vi "Write frame.vi"(8 "error in (no error)":errorcluster, 10 "frame":T1, 11 "Ephemeris in":refnum<class "Ephemeris.lvclass">) -> (0 "error out":errorcluster, 3 "Ephemeris out":refnum<class "Ephemeris.lvclass">)   [LabVIEW 2022 SP3, in "TCSDataDefinitions.lvlib" / "TCSCommand.lvlib" / "TargetConfiguration.lvlib" / "Target.lvlib" / "Ephemeris.lvclass"]
uses:
  Ephemeris.lvclass
  FixedTarget/Enumerations/FrameValues.ctl
  Ephemeris.lvclass/Ephemeris.ctl
  FixedTarget/FixedTarget.lvlib
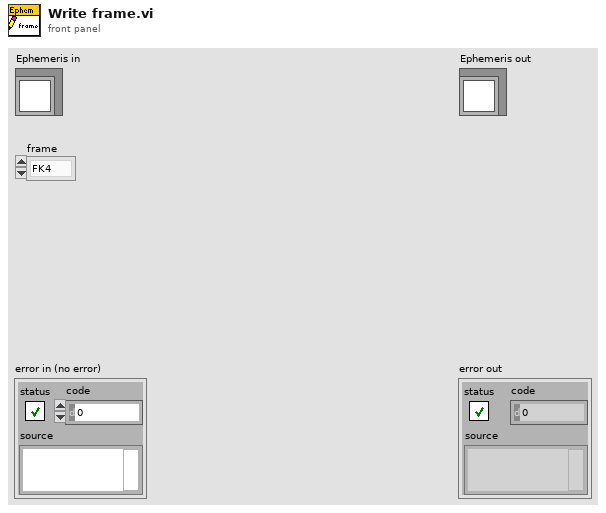
[diagram p1: front panel]
types:
  T1 = typedef "TCSDataDefinitions.lvlib/TCSCommand.lvlib/TargetConfiguration.lvlib/Target.lvlib/FixedTarget.lvlib/FrameValues.ctl" = enum16{"FK4", "FK5", "APPT", "GAPPT", "AZEL"}
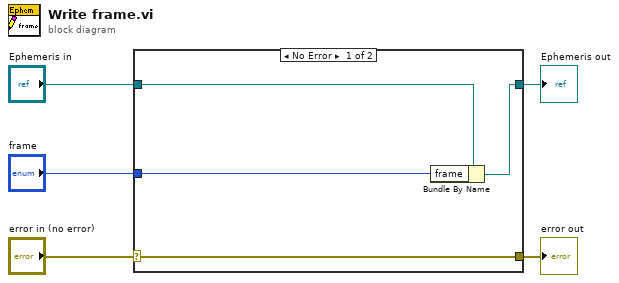
[diagram p0: block diagram]
diagram:
  n1 = case shown="No Error" "error in (no error)" {
    selector: "error in (no error)" -> [w9 w10]
    tunnel: [w9 w10] -> w4
    tunnel: [w7 w11] -> w2
    tunnel: "Ephemeris in" -> [w8 w11]
    tunnel: "frame" -> [w6 _]
    frame No Error {
      n2 = Bundle By Name(cluster=w8, "frame"=w6) -> (w7:refnum<class "Ephemeris.lvclass">)
    }
    frame Error {
    }
  }
  "error out" <- w4
  "Ephemeris out" <- w2
